vi "中值滤波.vi"() -> ()   [LabVIEW 2018]
uses:
  <vilib>/vision/NI_Vision_Development_Module.lvlib
panel:
  out "Image 2":T1(plugin-control)
  out "Image":T1(plugin-control)
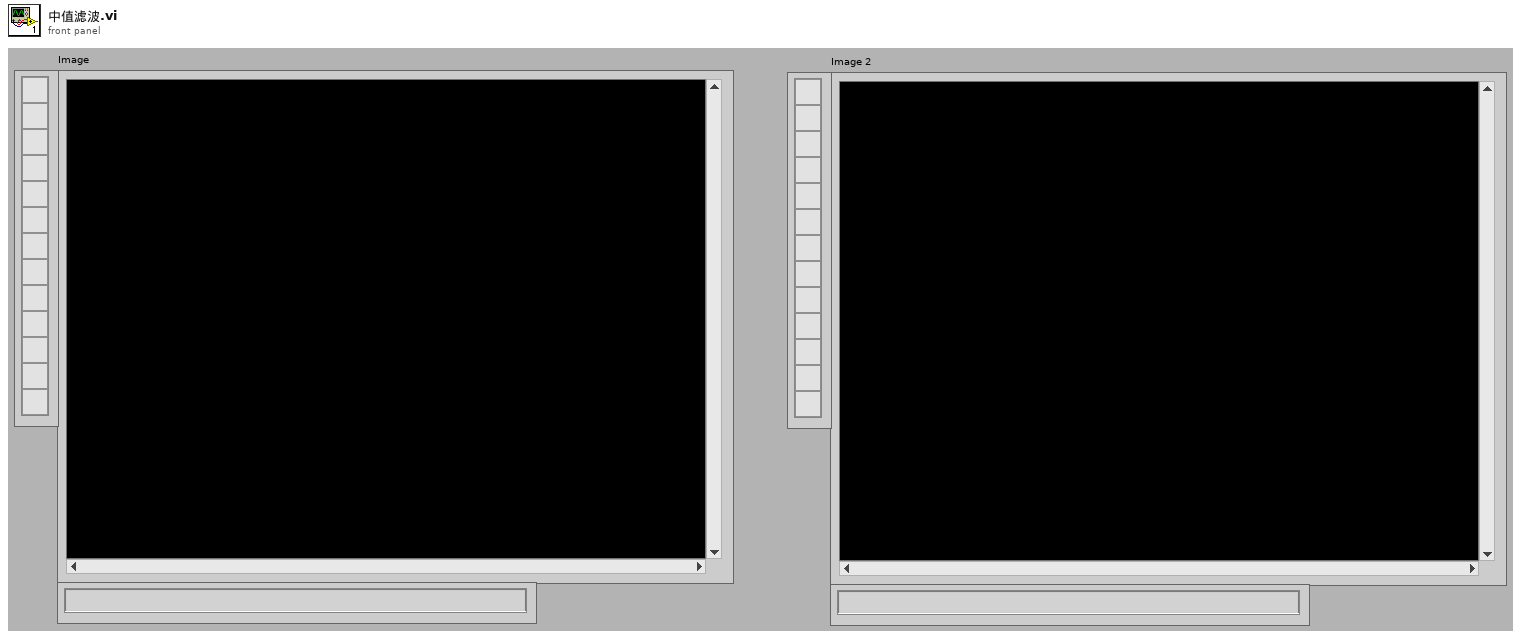
[diagram p1: front panel]
types:
  T1 = typedef "IMAQ Image.ctl" = refnum<image>
  T2 = typedef "Image Type" = u32
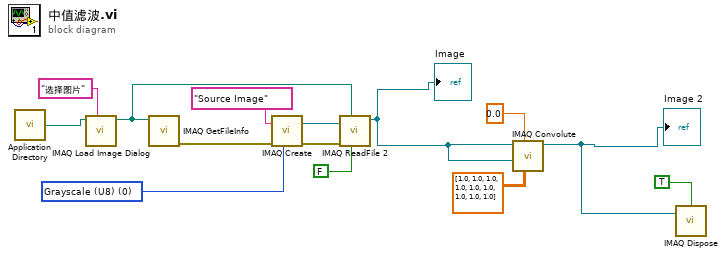
[diagram p0: block diagram]
diagram:
  w7 = T2 0 items=["Grayscale (U8)", "Grayscale (I16)", "Grayscale (SGL)", "Complex (CSG)", "RGB (U32)", "HSL (U32)", "RGB (U64)", "Grayscale (U16)"] ("Image Type")
  n1 = call <vilib>:"Application Directory.vi"() -> ("Application Directory"=w8:path)
  n2 = call "IMAQ Load Image Dialog"("Prompt"="选择图片" ("prompt"), "Start Path"=w8) -> ("Path"=w14:path)  [unwired: 7 in, 2 out]
  n3 = call "IMAQ GetFileInfo"("File Path"=w14) -> ("error out"=w12:errorcluster)  [unwired: 4 in, 6 out]
  n4 = call "IMAQ Create"("Image Name"="Source Image", "Image Type"=w7, "error in (no error)"=w12) -> ("New Image"=w10:T1, "error out"=w9:errorcluster)  [unwired: 2 in]
  n5 = call "IMAQ ReadFile 2"("Use File Path Image Type"=FALSE, "File Path"=w14, "error in (no error)"=w9, "Image"=w10) -> ("Image Out"=w1:T1)  [unwired: 3 in, 4 out]
  "Image" <- w1
  n6 = call "IMAQ Convolute"("Kernel"=sgl[][] [[1.0, 1.0, 1.0], [1.0, 1.0, 1.0], [1.0, 1.0, 1.0]], "Divider (kernel sum)"=sgl 0.0, "Image Dst"=w1, "Image Src"=w1) -> ("Image Dst Out"=w2:T1)  [unwired: 6 in, 1 out]
  "Image 2" <- w2
  n7 = call "IMAQ Dispose"("All Images? (No)"=TRUE, "Image"=w2) -> ()  [unwired: 1 in, 4 out]
